vi "Build JSON.vi"(8 "error in (no error)":errorcluster, 11 "Client Message in":refnum<class "Client Message.lvclass">) -> (0 "error out":errorcluster, 2 "JSON":string, 3 "Client Message out":refnum<class "Client Message.lvclass">)   [LabVIEW 2022 SP3, in "obs-websocket-lv.lvlib" / "Client Message.lvclass"]
uses:
  Client Message.lvclass
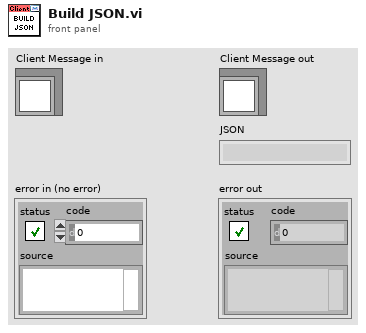
[diagram p1: front panel]
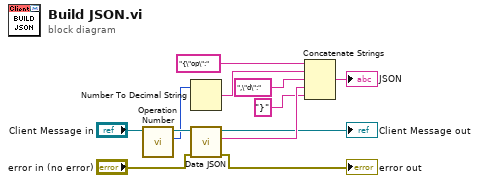
[diagram p0: block diagram]
diagram:
  n1 = call "Operation Number.vi"("Client Message in"="Client Message in") -> ("Operation Num"=w10:i32, "Client Message out"=w11:refnum<class "Client Message.lvclass">)  [unwired: 8 in, 1 out]
  n2 = Number To Decimal String(number=w10) -> (decimal integer string=w8:string)  [unwired: 1 in]
  n3 = call-dynamic "Data JSON.vi"("error in (no error)"="error in (no error)", "Client Message in"=w11) -> ("error out"=→"error out":errorcluster, "Data JSON"=w6:string, "Client Message out"=→"Client Message out":refnum<class "Client Message.lvclass">)  [unwired: 7 in]
  n4 = Concatenate Strings("{\"op\":" ("string"), w8, ",\"d\":" ("string"), w6, "}" ("string")) -> (→"JSON":string)
